vi "_initialDataPluginColumnListBoxes.vi"(8 "error in (no error)":errorcluster, 11 "MulticolumnListbox in":refnum<vi>) -> (0 "error out":errorcluster, 3 "MulticolumnListbox out":refnum<vi>)   [LabVIEW 2017]
uses:
  <vilib>/Utility/miscctls.llb/LVRowAndColumnTypeDef.ctl
  <vilib>/Utility/miscctls.llb/LVRowAndColumnUnsignedTypeDef.ctl
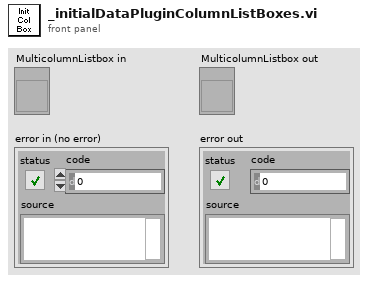
[diagram p1: front panel]
types:
  T1 = typedef "LVRowAndColumnUnsignedTypeDef.ctl" = cluster{"Row":u32, "Column":u32}
  T2 = typedef "LVRowAndColumnTypeDef.ctl" = cluster{"Row":i32, "Column":i32}
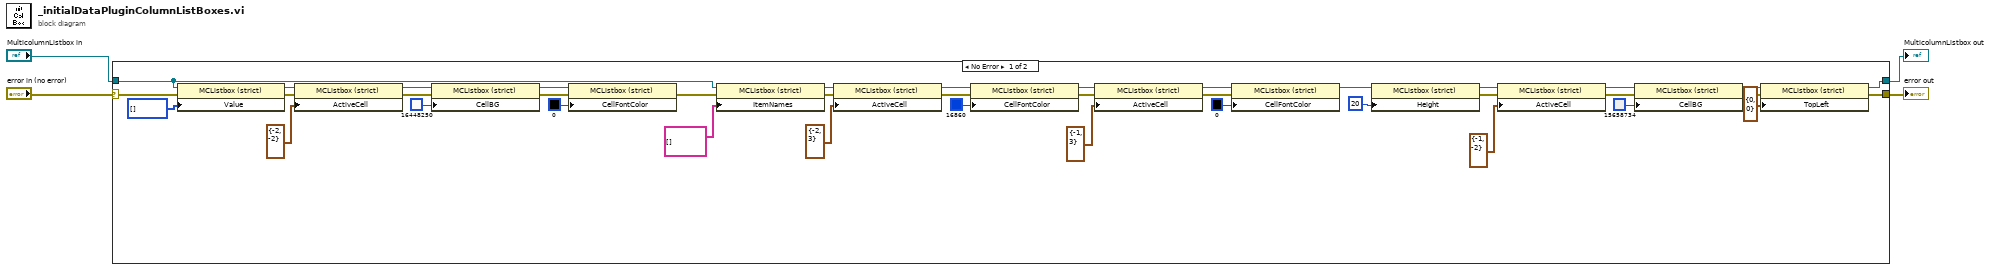
[diagram p0: block diagram]
diagram:
  n1 = case shown="No Error" "error in (no error)" {
    selector: "error in (no error)" -> [w10 w45]
    tunnel: "MulticolumnListbox in" -> [w38 w44]
    tunnel: [w8 w45] -> w3
    tunnel: [w7 w44] -> w1
    frame No Error {
      n2 = property class="MCListbox (strict)"(reference=w38, error in=w10, "Value"=i32[] []) -> (reference out=w29:refnum<vi>, error out=w30:errorcluster)
      n3 = property class="MCListbox (strict)"(reference=w29, error in=w30, "ActiveCell"=T2 {"Row"=-2, "Column"=-2} ("Active Cell:Active Cell")) -> (reference out=w22:refnum<vi>, error out=w26:errorcluster)
      n4 = property class="MCListbox (strict)"(reference=w22, error in=w26, "CellBG"=u32 16448250 ("Color Box")) -> (reference out=w24:refnum<vi>, error out=w27:errorcluster)
      n5 = property class="MCListbox (strict)"(reference=w24, error in=w27, "CellFontColor"=u32 0 ("Color Box")) -> (error out=w31:errorcluster)  [unwired: 1 out]
      n6 = property class="MCListbox (strict)"(reference=w38, error in=w31, "ItemNames"=string[][] [] ("Item Names")) -> (reference out=w43:refnum<vi>, error out=w39:errorcluster)
      n7 = property class="MCListbox (strict)"(reference=w43, error in=w39, "ActiveCell"=T2 {"Row"=-2, "Column"=3} ("Active Cell:Active Cell")) -> (reference out=w33:refnum<vi>, error out=w40:errorcluster)
      n8 = property class="MCListbox (strict)"(reference=w33, error in=w40, "CellFontColor"=u32 16860 ("Color Box")) -> (reference out=w35:refnum<vi>, error out=w41:errorcluster)
      n9 = property class="MCListbox (strict)"(reference=w35, error in=w41, "ActiveCell"=T2 {"Row"=-1, "Column"=3} ("Active Cell:Active Cell")) -> (reference out=w36:refnum<vi>, error out=w42:errorcluster)
      n10 = property class="MCListbox (strict)"(reference=w36, error in=w42, "CellFontColor"=u32 0 ("Color Box")) -> (reference out=w20:refnum<vi>)  [unwired: 1 out]
      n11 = property class="MCListbox (strict)"(reference=w20, "Height"=u32 20 ("Active Cell:Cell Size:Height")) -> (reference out=w16:refnum<vi>, error out=w12:errorcluster)  [unwired: 1 in]
      n12 = property class="MCListbox (strict)"(reference=w16, error in=w12, "ActiveCell"=T2 {"Row"=-1, "Column"=-2} ("Active Cell:Active Cell")) -> (reference out=w18:refnum<vi>, error out=w11:errorcluster)
      n13 = property class="MCListbox (strict)"(reference=w18, error in=w11, "CellBG"=u32 15658734 ("Color Box")) -> (reference out=w6:refnum<vi>, error out=w9:errorcluster)
      n14 = property class="MCListbox (strict)"(reference=w6, error in=w9, "TopLeft"=T1 {"Row"=0, "Column"=0} ("Top Left Visible Cell")) -> (reference out=w7:refnum<vi>, error out=w8:errorcluster)
    }
    frame Error {
    }
  }
  "error out" <- w3
  "MulticolumnListbox out" <- w1
